vi "Get Controls in Tab Control.vi"(8 "error in (no error)":errorcluster, 11 "TabCtl Ref":refnum<vi>) -> (0 "error out":errorcluster, 2 "Controls[]":refnum<vi>[](array[refnum]), 3 "TabCtl Ref out":refnum<vi>)   [LabVIEW 2022 SP3, in "MacroAssert.lvlib"]
doc: "Gets all control references within <B>TabCtl Ref</B> recursively by checking it for subpanels, getting any controls in them, checking for nested subpanels, etc."
uses:
  MacroAssert.lvlib
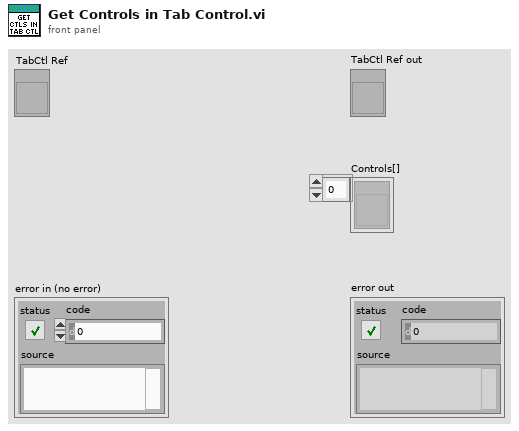
[diagram p1: front panel]
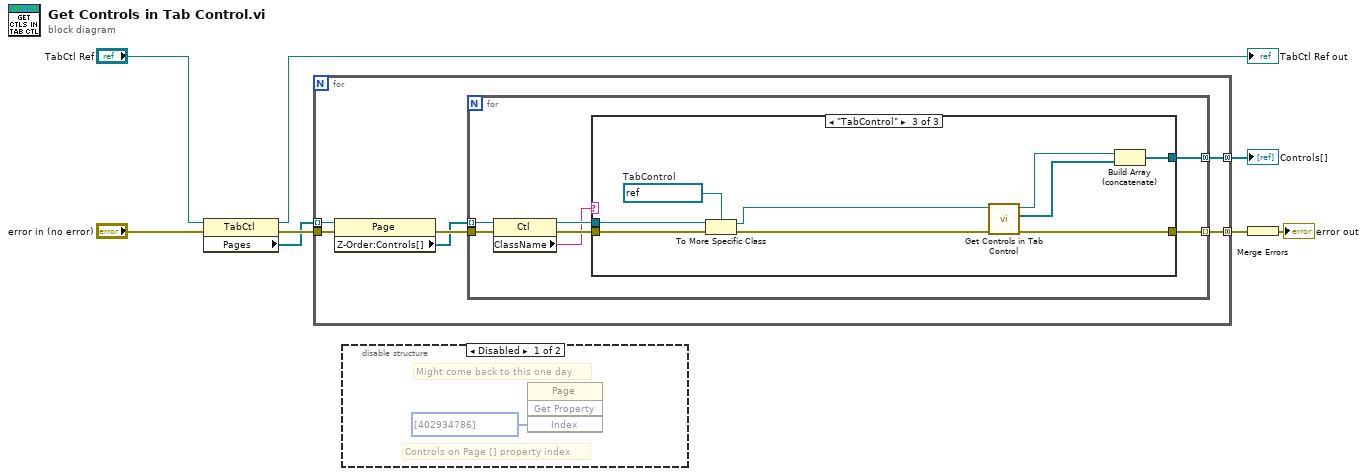
[diagram p0: block diagram]
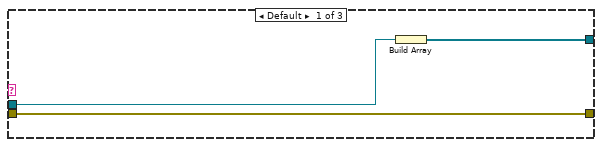
[diagram p3: hidden frame]
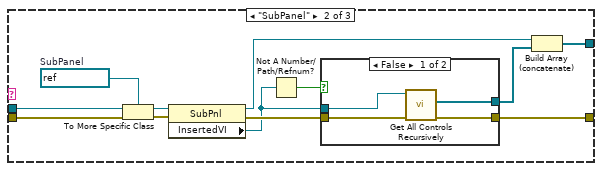
[diagram p4: hidden frame]
diagram:
  n1 = property class="TabCtl"(reference="TabCtl Ref", error in="error in (no error)") -> (reference out=→"TabCtl Ref out":refnum<vi>, error out=w7:errorcluster, "Pages"=w1:refnum<vi>[])
  n2 = for {
    tunnel: [w10] -> w2 mode=concatenating
    tunnel: w1 -> [w12] mode=indexing
    tunnel: w7 -> [w14]
    tunnel: [w11] -> w3 mode=concatenating
    n3 = property class="Page"(reference=w12, error in=w14) -> (error out=w13:errorcluster, "Z-Order:Controls[]"=w9:refnum<vi>[])  [unwired: 1 out]
    n4 = for {
      tunnel: [w16] -> w10 mode=concatenating
      tunnel: [w21] -> w11 mode=indexing
      tunnel: w13 -> [w19]
      tunnel: w9 -> [w17] mode=indexing
      n5 = property class="Ctl"(reference=w17, error in=w19) -> (reference out=w18:refnum<vi>, error out=w20:errorcluster, "ClassName"=w15:string)
      n6 = case shown="\"TabControl\"" w15 {
        tunnel: [w24 w33 w48] -> w21
        tunnel: w18 -> [w23 w30 w46]
        tunnel: w20 -> [w24 w36 w50]
        tunnel: [w22 w26 w43] -> w16
        frame Default {
          n7 = Build Array(w23) -> (w22:refnum<vi>[])
        }
        frame "SubPanel" {
          w31 = refnum<vi> refnum  # SubPanel
          n8 = To More Specific Class(target class=w31, reference=w30, error in=w36) -> (specific class reference=w32:refnum<vi>, error out=w35:errorcluster)
          n9 = property class="SubPnl"(reference=w32, error in=w35) -> (reference out=w29:refnum<vi>, error out=w34:errorcluster, "InsertedVI"=w28:refnum<vi>)
          n10 = Not A Number/Path/Refnum?(number/path/refnum=w28) -> (NaN/Path/Refnum?=w25:bool)
          n11 = case shown="False" w25 {
            tunnel: w34 -> [w40 w41]
            tunnel: [w39 w41] -> w33
            tunnel: [w37 _] -> w27
            tunnel: w28 -> [w38 _]
            frame False {
              n12 = call "Get All Controls Recursively.vi"("error in (no error)"=w40, "VI Ref"=w38) -> ("error out"=w39:errorcluster, "Controls[]"=w37:refnum<vi>[])  [unwired: 7 in, 1 out]
            }
            frame True {
            }
          }
          n13 = Build Array (concatenate)(w29, w27) -> (w26:refnum<vi>[])
        }
        frame "TabControl" {
          w47 = refnum<vi> refnum  # TabControl
          n14 = To More Specific Class(target class=w47, reference=w46, error in=w50) -> (specific class reference=w45:refnum<vi>, error out=w49:errorcluster)
          n15 = call "Get Controls in Tab Control.vi"("error in (no error)"=w49, "TabCtl Ref"=w45) -> ("error out"=w48:errorcluster, "Controls[]"=w42:refnum<vi>[], "TabCtl Ref out"=w44:refnum<vi>)  [unwired: 7 in]
          n16 = Build Array (concatenate)(w44, w42) -> (w43:refnum<vi>[])
        }
      }
    }
  }
  "Controls[]" <- w2
  n17 = disable-structure shown="Disabled" {
    frame Disabled {
      # "Might come back to this one day"
      # "Controls on Page [] property index"
      n18 = invoke class="Page" method="Get Property"("Index"=i32[] [402934786]) -> ()  [unwired: 3 in, 4 out]
    }
    frame Enabled {
    }
  }
  n19 = Merge Errors(w3) -> (→"error out":errorcluster)
